vi "DAQ_Manager.DAQ_Manager.setDAQConfig.vi"(8 "error in (no error)":errorcluster, 10 "DAQ_Manager.setDAQConfig":T1 {"DAQmx.AI.config"."input terminal configuration" items=["default"=-1, "RSE"=10083, "NRSE"=10078, "Differential"=10106, "Pseudodifferential"=12529]; "DAQmx.AI.config"."AI.Coupling" items=["AC"=10045, "DC"=10050, "GND"=10066]; "DAQmx.AO.config"."output terminal configuration" items=["Default"=-1, "RSE"=10083, "Differential"=10106, "Pseudodifferential"=12529]}, 11 "DAQ_Manager":refnum<class "DAQ_Manager.lvclass">) -> (0 "error out":errorcluster, 3 "DAQ_Manager out":refnum<class "DAQ_Manager.lvclass">)   [LabVIEW 2016, in "DAQ_Manager.lvclass"]
doc: "---------------------------------------------------------------\nJKI State Machine Objects™\nhttp://jki.net/state-machine-objects/\nCopyright (C) 2005-2015, JKI <info@jki.net>\nALL RIGHTS RESERVEDJKI State Machine Objects (SMO) 1.0.0.4\nJKI - JKI\nCopyright (c) 2015, JKI"
uses:
  DAQ_Manager.lvclass
  Typedefs/PrivateEvents--DAQ_Manager.DAQ_Manager.setDAQConfig.ctl
  DAQmx.AI/Typedefs/DAQmx.AI_Config.ctl
  DAQmx.AI/Typedefs/AI.Coupling-enum.ctl
  DAQmx.AI/Typedefs/AI.Terminal-enum.ctl
  DAQmx.AO/Typedefs/DAQmx.AO_Config.ctl
  DAQmx.AO/Typedefs/AO.Terminal-enum.ctl
  DAQ_Manager.lvclass/DAQ_Manager.ctl
  DAQmx.AO/DAQmx.AO.lvclass
  DAQmx.AI/DAQmx.AI.lvclass
panel:
  # "For instructions on how to use the JKI State Machine Objects, examples and video tutorials, visit:\nhttp://jki.net/state-machine-objects/\n\nJKI State Machine Objects™\nhttp://jki.net/state-machine-objects/\nCopyright (C) 2005-2015, JKI <info@jki.net>\nALL RIGHTS RESERVED"
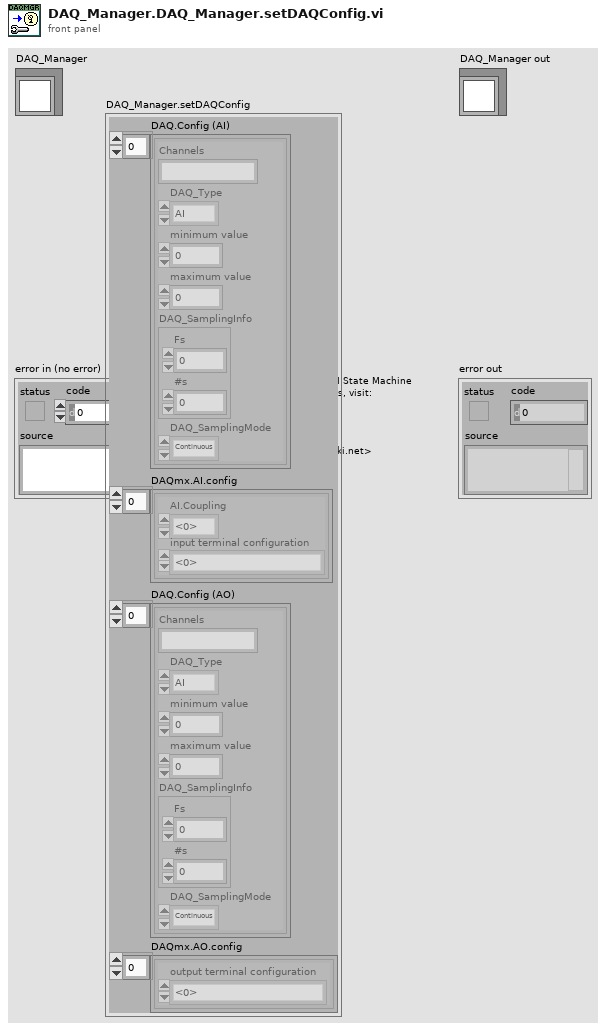
[diagram p1: front panel]
types:
  T1 = typedef "DAQ_Manager.lvclass/PrivateEvents--DAQ_Manager.DAQ_Manager.setDAQConfig.ctl" = cluster{"DAQ.Config (AI)":cluster{"Channels":string, "DAQ_Type":enum16{"AI", "AO"}, "minimum value":dbl, "maximum value":dbl, "DAQ_SamplingInfo":cluster{"Fs":dbl, "#s":i32}, "DAQ_SamplingMode":enum16{"Continuous", "Finite"}}[], "DAQmx.AI.config":T2[], "DAQ.Config (AO)":cluster{"Channels":string, "DAQ_Type":enum16{"AI", "AO"}, "minimum value":dbl, "maximum value":dbl, "DAQ_SamplingInfo":cluster{"Fs":dbl, "#s":i32}, "DAQ_SamplingMode":enum16{"Continuous", "Finite"}}[], "DAQmx.AO.config":T5[]}
  T2 = typedef "DAQmx.AI.lvclass/DAQmx.AI_Config.ctl" = cluster{"AI.Coupling":T3, "input terminal configuration ":T4}
  T3 = typedef "DAQmx.AI.lvclass/AI.Coupling-enum.ctl" = i32
  T4 = typedef "DAQmx.AI.lvclass/AI.Terminal-enum.ctl" = i32
  T5 = typedef "DAQmx.AO.lvclass/DAQmx.AO_Config.ctl" = cluster{"output terminal configuration":T6}
  T6 = typedef "DAQmx.AO.lvclass/AO.Terminal-enum.ctl" = i32
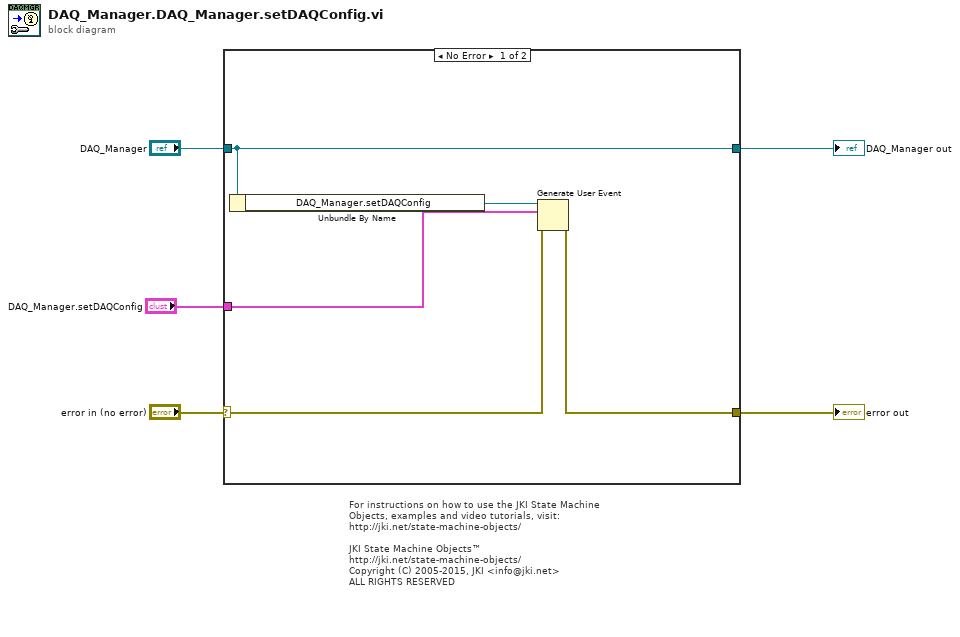
[diagram p0: block diagram]
diagram:
  # "For instructions on how to use the JKI State Machine Objects, examples and video tutorials, visit:\nhttp://jki.net/state-machine-objects/\n\nJKI State Machine Objects™\nhttp://jki.net/state-machine-objects/\nCopyright (C) 2005-2015, JKI <info@jki.net>\nALL RIGHTS RESERVED"
  n1 = case shown="No Error" "error in (no error)" {
    selector: "error in (no error)" -> [w10 w12]
    tunnel: [w7 w12] -> w4
    tunnel: [w6 w11] -> w5
    tunnel: "DAQ_Manager" -> [w6 w11]
    tunnel: "DAQ_Manager.setDAQConfig" -> [w9 _]
    frame No Error {
      n2 = Unbundle By Name(w6) -> ("DAQ_Manager.setDAQConfig"=w8:refnum<user-event>)
      n3 = Generate User Event(user event=w8, event data cluster=w9, error in=w10) -> (error out=w7:errorcluster)  [unwired: 1 in, 1 out]
    }
    frame Error {
    }
  }
  "error out" <- w4
  "DAQ_Manager out" <- w5
